vi "Testa_Leaf.vi"(9 "enable":bool, 11 "LEAF":i32) -> ()   [LabVIEW 2018]
uses:
  Global_Telescopio.vi
panel:
  out "error out 4":errorcluster
  out "error out 3":errorcluster
  out "error out 2":errorcluster
  out "concatenated string":string
  out "error out":errorcluster
  out "vi reference":refnum<vi>
  out "timeout":timestamp
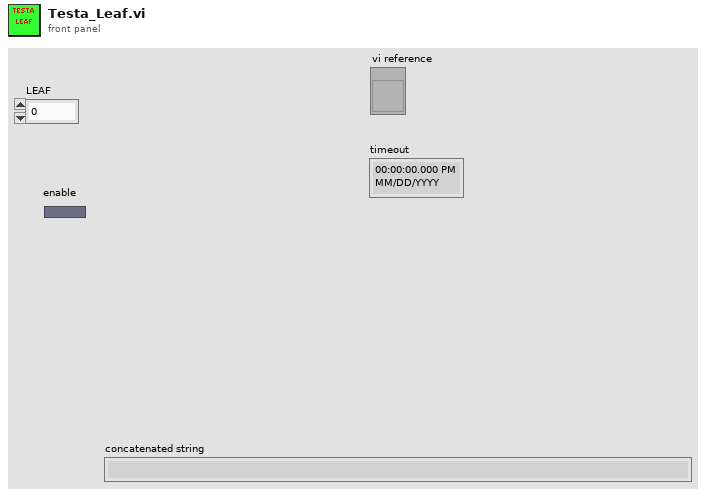
[diagram p1: front panel]
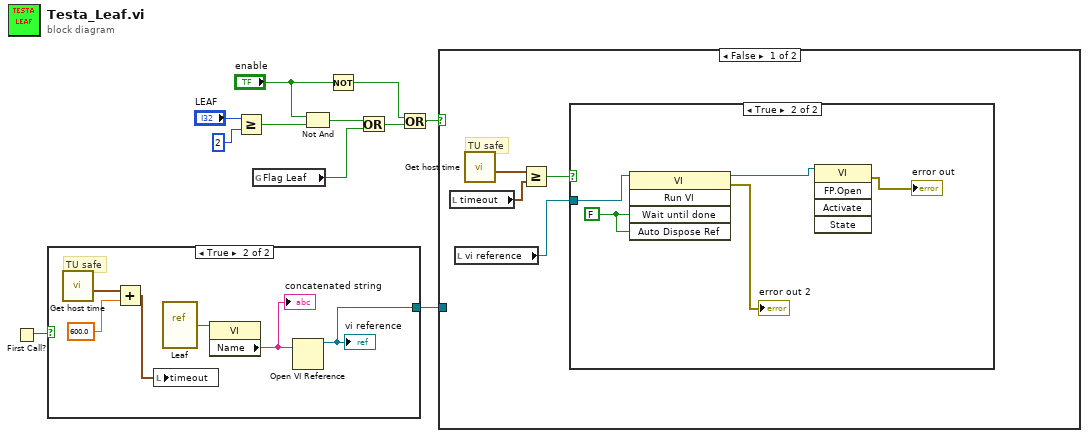
[diagram p0: block diagram]
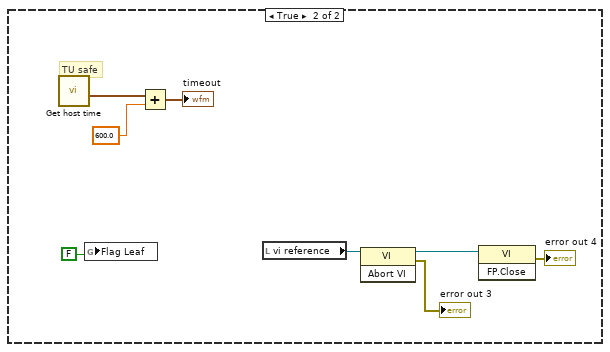
[diagram p4: hidden frame]
diagram:
  n1 = First Call?() -> (First Call?: T/F=w11:bool)
  n2 = case shown="True" w11 {
    tunnel: [_ w15] -> w10
    frame False {
    }
    frame True {
      # "TU safe"
      n3 = call "Get host time.vi"() -> ("BR current time"=w12:timestamp)  [unwired: 8 in, 3 out]
      n4 = Add(x=w12, y=600.0) -> (x+y=w13:timestamp)
      n5 = local write "timeout"(w13) -> ()
      n6 = vi-ref "Leaf.vi"() -> (w17:refnum<vi>)
      n7 = property class="VI"(reference=w17) -> ("Name"=w16:string)  [unwired: 1 in, 2 out]
      "concatenated string" <- w16
      n8 = Open VI Reference(vi path=w16) -> (vi reference=w15:refnum<vi>)  [unwired: 5 in, 1 out]
      "vi reference" <- w15
    }
  }
  n9 = Greater Or Equal?(x="LEAF", y=2) -> (x >= y?=w7:bool)
  n10 = global read "Global_Telescopio.vi" "Flag Leaf"() -> (w5:bool)
  n11 = Not And(1:w7, 2:"enable") -> (0:w6:bool)
  n12 = Not(x="enable") -> (.not. x?=w1:bool)
  n13 = Or(x=w6, y=w5) -> (x .or. y?=w4:bool)
  n14 = Or(x=w1, y=w4) -> (x .or. y?=w2:bool)
  n15 = case shown="False" w2 {
    tunnel: w10 -> [_ _]
    frame False {
      # "TU safe"
      n16 = local read "timeout"() -> (w21:timestamp)
      n17 = local read "vi reference"() -> (w20:refnum<vi>)
      n18 = call "Get host time.vi"() -> ("BR current time"=w18:timestamp)  [unwired: 8 in, 3 out]
      n19 = Greater Or Equal?(x=w18, y=w21) -> (x >= y?=w19:bool)
      n20 = case shown="True" w19 {
        tunnel: w20 -> [_ w25]
        frame False {
        }
        frame True {
          w26 = FALSE ("Wait Until Done")
          n21 = invoke class="VI" method="Run VI"(reference=w25, "Wait until done"=w26, "Auto Dispose Ref"=w26) -> (reference out=w24:refnum<vi>, error out=→"error out 2":errorcluster)  [unwired: 2 in, 3 out]
          n22 = invoke class="VI" method="FP.Open"(reference=w24) -> (error out=→"error out":errorcluster)  [unwired: 4 in, 4 out]
        }
      }
    }
    frame True {
      # "TU safe"
      n23 = call "Get host time.vi"() -> ("BR current time"=w27:timestamp)  [unwired: 8 in, 3 out]
      n24 = global write "Global_Telescopio.vi" "Flag Leaf"(FALSE) -> ()
      n25 = Add(x=w27, y=600.0) -> (x+y=→"timeout":timestamp)
      n26 = local read "vi reference"() -> (w30:refnum<vi>)
      n27 = invoke class="VI" method="Abort VI"(reference=w30) -> (reference out=w32:refnum<vi>, error out=→"error out 3":errorcluster)  [unwired: 2 in, 1 out]
      n28 = invoke class="VI" method="FP.Close"(reference=w32) -> (error out=→"error out 4":errorcluster)  [unwired: 2 in, 2 out]
    }
  }
